vi "getHWIO_1_exposureTrigger.vi"(8 "error in (no error)":errorcluster, 11 "Camera in":refnum<class "Camera.lvclass">) -> (0 "error out":errorcluster, 1 "polarity":u16(ring)=4 items=["rising edge"=4, "falling edge"=8], 2 "on":bool=TRUE, 3 "Camera out":refnum<class "Camera.lvclass">)   [LabVIEW 2019, in "Camera.lvclass"]
doc: "Gets HWIO exposure trigger polarity and status (enabled / disabled). Generates an error if camera is recording or if HWIO configuration is not supported."
uses:
  Camera.lvclass
  pco.sdk/TimingControl/TimingControl.lvlib
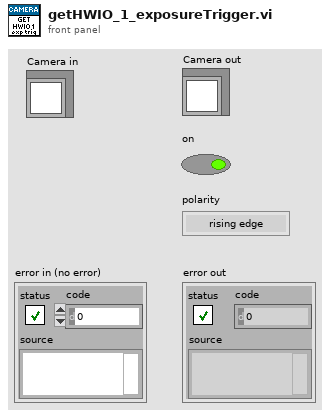
[diagram p1: front panel]
types:
  T1 = cluster{"wSignalNum":u16, "wEnabled":u16, "wType":u16, "wPolarity":u16, "wFilterSetting":u16, "wSelected":u16, "dwParameter":u32[], "dwSignalFunctionality":u32[]}
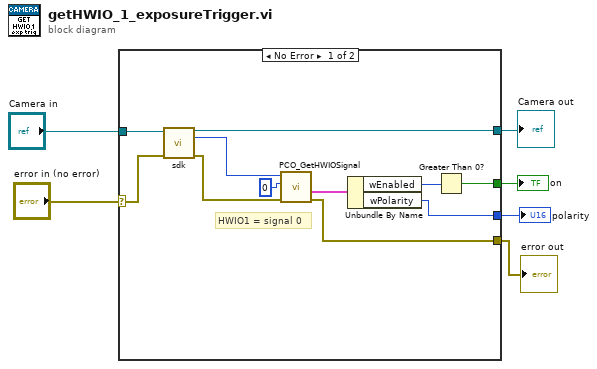
[diagram p0: block diagram]
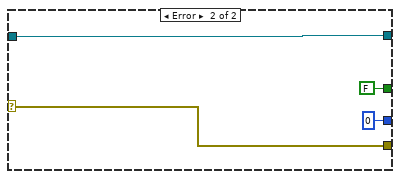
[diagram p2: hidden frame]
diagram:
  n1 = case shown="No Error" "error in (no error)" {
    selector: "error in (no error)" -> [w11 w18]
    tunnel: "Camera in" -> [w16 w21]
    tunnel: [w14 w21] -> w4
    tunnel: [w12 w18] -> w1
    tunnel: [w8 FALSE] -> w3
    tunnel: [w7 u16 0 ("wPolarity")] -> w2
    frame No Error {
      # "HWIO1 = signal 0"
      n2 = call-dynamic "sdk.vi"("Camera in"=w16, "error in (no error)"=w11) -> ("Camera out"=w14:refnum<class "Camera.lvclass">, "sdk"=w15:u64, "error out"=w10:errorcluster)  [unwired: 11 in]
      n3 = call "PCO_GetHWIOSignal.vi"("error in (no error)"=w10, "wSignalNum"=u16 0, "ph"=w15) -> ("error out"=w12:errorcluster, "strSignal"=w13:T1)  [unwired: 5 in, 2 out]
      n4 = Unbundle By Name(w13) -> ("wEnabled"=w9:u16, "wPolarity"=w7:u16)
      n5 = Greater Than 0?(x=w9) -> (x > 0?=w8:bool)
    }
    frame Error {
    }
  }
  "Camera out" <- w4
  "error out" <- w1
  "on" <- w3
  "polarity" <- w2
